vi "Auto Catapult Mode.vi"(9 "Ball Loaded?":bool, 10 "Limit Switch Activated?":bool, 11 "Catapult Commands":T1={"Command"=enum."Prime Shooter", "Mode"=enum."Manual", "Override Trigger Sensor"=FALSE, "High Power Shot?"=FALSE, "Vision?"=FALSE}) -> (0 "Secure Ball?":bool, 1 "Pinned?":bool, 2 "Low Power Solenoid":bool, 3 "High Power Solenoid":bool)   [LabVIEW 2015]
uses:
  Common Code/Catapult/Catapult Command Cluster.ctl
  Common Code/Shooter Commands.ctl
  Common Code/Shoot Modes Enum.ctl
  Common Code/Catapult/Catapult State.ctl
  Common Code/Change Detect Boolean.vi
  Common Code/Change Detect Int.vi
  Robot Global Data.vi
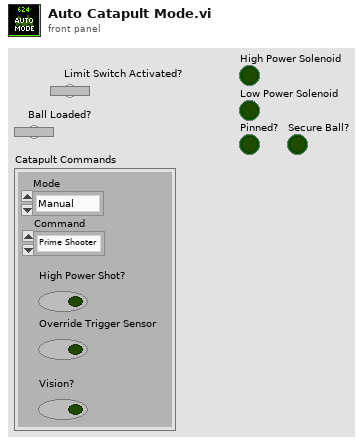
[diagram p1: front panel]
types:
  T1 = typedef "Catapult Command Cluster.ctl" = cluster{"Command":T2, "Mode":T3, "Override Trigger Sensor":bool, "High Power Shot?":bool, "Vision?":bool}
  T2 = typedef "Shooter Commands.ctl" = enum16{"Idle", "Prime Shooter", "Shoot"}
  T3 = typedef "Shoot Modes Enum.ctl" = enum16{"Manual", "Safe", "Auto"}
  T4 = typedef "Catapult State.ctl" = enum16{"Idle", "Warmup", "Shooter Ready", "Shoot"}
  T5 = typedef "Intake Status Cluster.ctl" = cluster{"Roller Power":dbl, "Angle Power":dbl, "Intake Mode":T6, "Intake States":T7, "Rollers Active?":bool, "Current Height":dbl, "Target Height":dbl, "Encoder Raw Position":dbl, "Forward Tripped?":bool, "Backward Tripped?":bool, "Override IR?":bool}
  T6 = typedef "Intake Mode.ctl" = enum16{"Safe", "Auto", "Manual"}
  T7 = typedef "Intake States.ctl" = enum16{"Idle", "Set roller speed", "Move to angle", "Go Hard or Go Home", "Ball Settle"}
  T8 = typedef "Drivetrain Status Cluster.ctl" = cluster{"Modes":T9, "Y (Throttle)":dbl, "X (Steer)":dbl, "Gyro In Range?":bool, "Distance Drive Finished?":bool, "Stop Eject Lockout":bool, "Dist Drive Status":T10, "Y Target":dbl, "Heading Target":dbl, "Vision Target Aligned?":bool, "Gear":dbl, "1st Gear Time":dbl, "2nd Gear Time":dbl, "1st Gear Shifts":dbl, "2nd Gear Shifts":dbl}
  T9 = typedef "Drivetrain Modes.ctl" = enum16{"Tank", "Climb", "Manual", "Goal Vision Targeting", "PID Distance Drive", "Hybrid", "Gyro Steer"}
  T10 = typedef "Dist Drive Status.ctl" = cluster{"Y In Range":bool, "X In Range":bool, "Gyro In Range":bool, "Y Dist":dbl, "X Dist":dbl, "Gyro":dbl}
  T11 = typedef "Dashboard Control Data.ctl" = cluster{"Shooter Presets":T12, "Encoder Control":T14, "Steer PID output":cluster{"output high":dbl, "output low":dbl}, " Steer PID gains":cluster{"proportional gain (Kc)":dbl, "integral time (Ti, min)":dbl, "derivative time (Td, min)":dbl}, "Drivetrain Settings":T15, "Vision Packet":T16, "Dashboard Drivetrain Command":T17, "Info/Command Cluster":T19, "Ball Vision Packet":T20, "Intake Presets":T22, "Intake Encoder Control":T24, "Climb Presets":T25, "Goal Output Range":cluster{"output high":dbl, "output low":dbl}, "Enabled Systems":T26, "Auton Presets":T27, "Pressure M":dbl, "Pressure B":dbl, "Vision Timeout":dbl, "Auto-Shift":T28, "Catapult Setpoints":T29}
  T12 = typedef "Shooter Presets.ctl" = cluster{"Batter Shot":T13, "Deep Middle":T13, "Manual Shot":T13, "Left Ticks Per Rotation":dbl, "Right Ticks Per Rotation":dbl, "Low Bar Shot":T13, "Shooter RPM Tolerance":dbl, "Trigger Power":dbl, "Fire from Load Delay":i32, "Max Angle":dbl, "Min Angle":dbl, "Angle PID gains":cluster{"P":dbl, "I":dbl, "D":dbl}, "Angle Output":cluster{"output high":dbl, "output low":dbl}, "Shooter Angle Tolerance":dbl, "Vision Shoot x^2":dbl, "Vision Shoot x":dbl, "Feed Forward Max Accel":dbl, "Feed Forward Kv":dbl, "Backwards Trigger":dbl, "Shot Finish Delay (ms)":dbl, "Angle Max Current":dbl, "Angle Current Trip Time":dbl, "Intake Angle":dbl, "Vision Shoot c":dbl, "Reset?":bool, "Button Release Delay":dbl, "Angle Pot x":dbl, "Angle Pot c":dbl, "Ignore Angle?":bool, "Max RPM":dbl, "Safty Frist Angle":dbl, "Intake Danger Height":dbl, "Angle Pot B":i32, "Angle Pot M":dbl, "FF Finish RPM":dbl, "RPM PID Right":cluster{"P":dbl, "I":dbl, "D":dbl, "FF":dbl}, "RPM PID Left":cluster{"P":dbl, "I":dbl, "D":dbl, "FF":dbl}, "Backwards RPM":dbl, "Vision RPM":dbl, "Run Wheels Backward Delay":u32, "Cleat Shot":T13, "Vision Far RPM":dbl, "Vision Far Distance":dbl, "Vision Far Angle":dbl}
  T13 = typedef "Shot Presets.ctl" = cluster{"L":dbl, "R":dbl, "A":dbl}
  T14 = typedef "Encoder Control.ctl" = cluster{"Right Tick Constant":dbl, "Left Tick Constant":dbl, "Reset?":bool, "Y Dist":cluster{"PID gains":cluster{"proportional gain (Kc)":dbl, "integral time (Ti, min)":dbl, "derivative time (Td, min)":dbl}}, "Y Stop Thresh":dbl, "Y Stop Speed":dbl}
  T15 = typedef "Drivetrain Settings.ctl" = cluster{"Gyro Tolerance":dbl, "Throttle Ramp (ms)":dbl, "Kv":dbl, "Ka":dbl, "Feed Forward P":dbl, "Feed Forward D":dbl, "Goal Vision PID gains":cluster{"proportional gain (Kc)":dbl, "integral time (Ti, min)":dbl, "derivative time (Td, min)":dbl}, "Goal Detection Window":dbl, "Creep Rate":dbl, "Vision Throttle Threshold":dbl, "Min Turn Output":dbl, "Left Batter Angle":dbl, "Right Batter Angle":dbl}
  T16 = typedef "Goal Vision Packet.ctl" = cluster{"Distance":dbl, "Center X":dbl, "Center Y":dbl, "Found Target?":bool, "Robot Center":dbl, "Angle":dbl}
  T17 = typedef "Dashboard Drivetrain Command.ctl" = cluster{"Drivetrain Vision":T18}
  T18 = typedef "Drivetrain Vision.ctl" = cluster{"Goal Window":dbl, "Ball Window":dbl}
  T19 = typedef "Ball Tracking Command Cluster.ctl" = cluster{"Distance to Ball":dbl, "Desired Angle":dbl, "Command":enum16{"Turn to Ball", "Turn to Angle", "Get Distance"}, "Pixels from Center":dbl}
  T20 = typedef "Ball Vision Packet.ctl" = cluster{"Ball Detected?":bool, "Distance to Ball":dbl, "Desired Angle":dbl, "Pixels from Center":dbl, "Tracking mode":T21}
  T21 = typedef "Tracking Mode.ctl" = enum16{"Turn to Ball", "Turn to Angle"}
  T22 = typedef "Intake Presets.ctl" = cluster{"Intake Speed":dbl, "Outake Speed":dbl, "Low Height":dbl, "Half Height":dbl, "High Idle Height":dbl, "Angle Speed":dbl, "Angle Tolerance":dbl, "Encoder Scale":dbl, "Load Height":dbl, "Output Range":T23, "Rotation Power Max/Min":dbl, "MaxCurrent":dbl, "Intake Trip Time":dbl, "Idle Height":dbl, "Max Height":dbl, "Reset Encoders?":bool, "PID gains":cluster{"proportional gain (Kc)":dbl, "integral time (Ti, min)":dbl, "derivative time (Td, min)":dbl}, "Intake Stop Delay":u32, "Settle Time":dbl, "Settle Wait Time":dbl, "Pull Up Delay":dbl}
  T23 = typedef "Drivetrain Output Range.ctl" = cluster{"output high":dbl, "output low":dbl}
  T24 = typedef "IntakeEcoderControl.ctl" = cluster{"Arm Tick Constant":dbl, "Reset?":bool, "Y Dist":cluster{"PID gains":cluster{"proportional gain (Kc)":dbl, "integral time (Ti, min)":dbl, "derivative time (Td, min)":dbl}}, "Y Stop Thresh":dbl, "Y Stop Speed":dbl}
  T25 = typedef "Climb Presets.ctl" = cluster{"Pull Power":dbl, "Extend Power":dbl}
  T26 = typedef "Enabled Systems.ctl" = cluster{"Shoot":bool, "Intake":bool, "DT":bool, "Gyro":bool, "100ms":bool, "US":bool}
  T27 = typedef "Autonomous Presets.ctl" = cluster{"Pitch Limit":dbl, "Roll Limit":dbl, "Start Position":dbl, "Cross Position":dbl}
  T28 = typedef "Auto Shift Cluster.ctl" = cluster{"Delay":dbl, "Speed Thresh":dbl, "Upshift Accel":dbl, "Upshift Throttle":dbl, "Upshift Throttle Accel":dbl, "Downshift Throttle":dbl, "Downshift Throttle Accel":dbl, "Pressure Threshold":dbl}
  T29 = typedef "Catapult Setpoints.ctl" = cluster{"Intake Danger Height":dbl, "Claw Release Delay":dbl, "Shot Finish Delay":dbl, "Limit Switch Pin Delay":dbl}
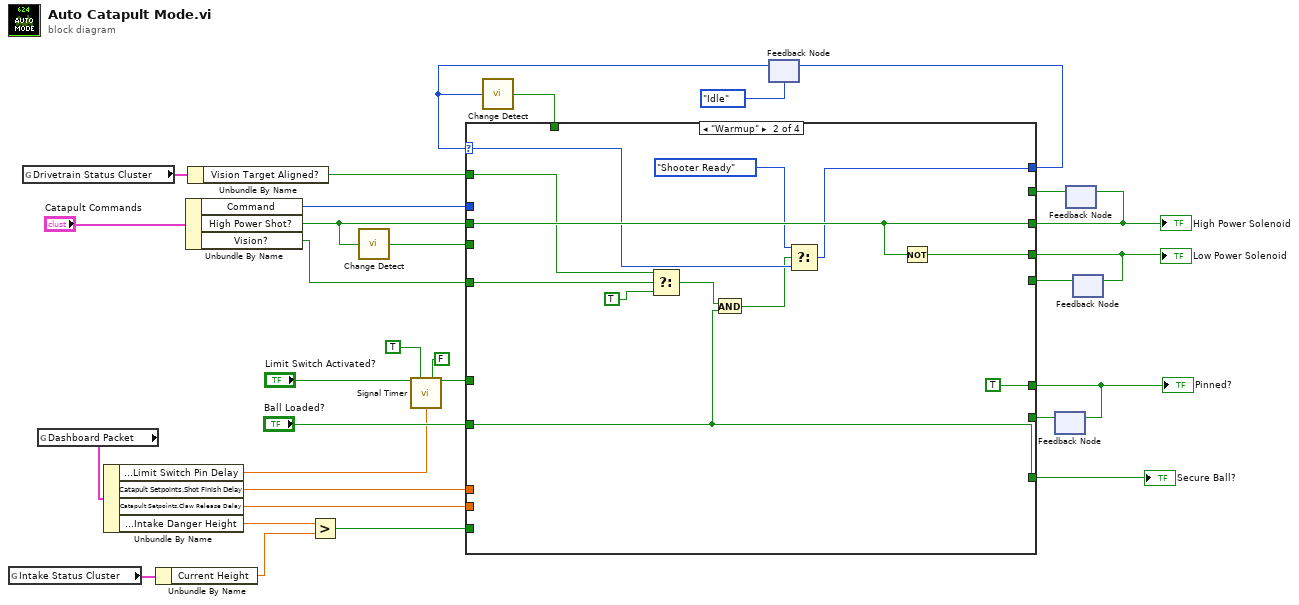
[diagram p0: block diagram]
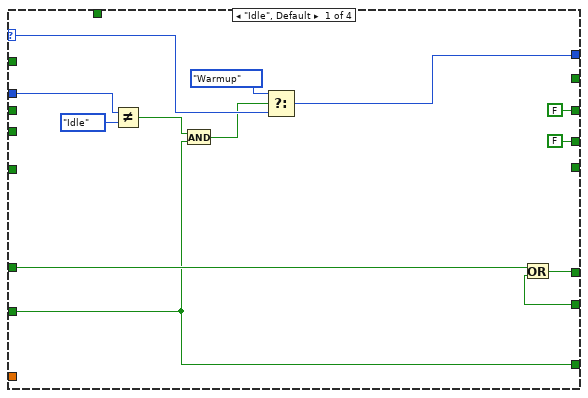
[diagram p2: hidden frame]
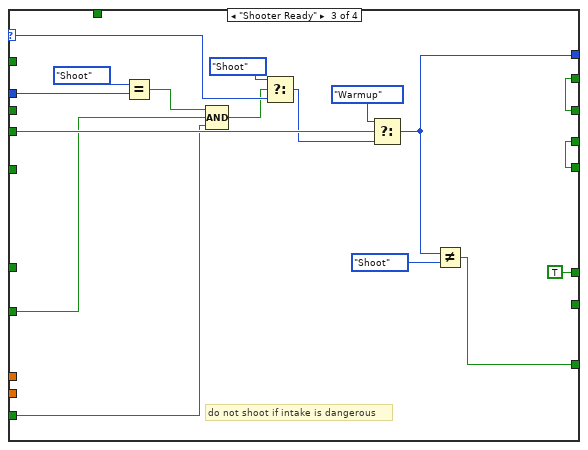
[diagram p3: hidden frame]
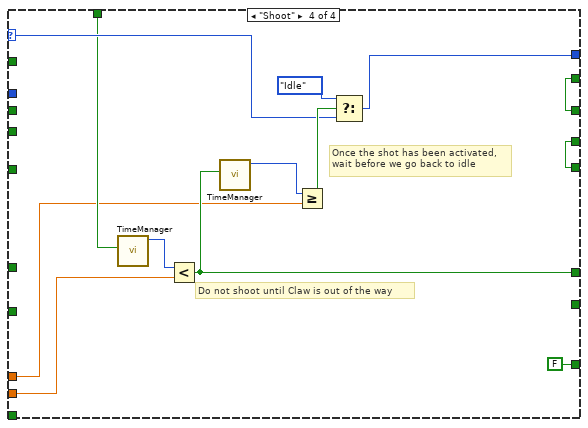
[diagram p4: hidden frame]
diagram:
  n1 = global read "Robot Global Data.vi" "Intake Status Cluster"() -> (w5:T5)
  n2 = global read "Robot Global Data.vi" "Drivetrain Status Cluster"() -> (w13:T8)
  n3 = global read "Robot Global Data.vi" "Dashboard Packet"() -> (w9:T11)
  n4 = Unbundle By Name(w9) -> ("Catapult Setpoints.Limit Switch Pin Delay"=w8:dbl, "Catapult Setpoints.Shot Finish Delay"=w7:dbl, "Catapult Setpoints.Claw Release Delay"=w6:dbl, "Catapult Setpoints.Intake Danger Height"=w4:dbl)
  n5 = Unbundle By Name(w5) -> ("Current Height"=w3:dbl)
  n6 = Unbundle By Name("Catapult Commands") -> ("Command"=w31:T2, "High Power Shot?"=w18:bool, "Vision?"=w14:bool)
  n7 = Unbundle By Name(w13) -> ("Vision Target Aligned?"=w12:bool)
  n8 = Greater?(x=w4, y=w3) -> (0:w2:bool)
  n9 = call-poly "Change Detect.vi"("In"=w18) -> ("Changed?"=w17:bool)
  n10 = call "Signal Timer.vi"("Input"="Limit Switch Activated?", "Edge"=TRUE, "Interval"=w8, "Pull"=FALSE) -> ("Filtered Output"=w21:bool)  [unwired: 11 in]
  n11 = feedback #1(Catapult_State."Idle") -> (w16:T4)
  n12 = call-poly "Change Detect.vi"("In"=w16) -> ("Changed?"=w15:bool)
  n13 = feedback #2() -> (w19:bool)  [unwired: 1 in]
  n14 = feedback #3() -> (w25:bool)  [unwired: 1 in]
  n15 = feedback #4() -> (w27:bool)  [unwired: 1 in]
  n16 = case shown="\"Warmup\"" w16 {
    selector: w16 -> [w42 w48 w68 w82]
    tunnel: w31 -> [w44 _ w70 _]
    tunnel: [w40 w49 w63 w80] -> w29
    tunnel: w18 -> [_ w56 _ _]
    tunnel: [FALSE ("High Power Shot?") w56 w71 w86] -> w26
    tunnel: [FALSE w55 w72 w85] -> w28
    tunnel: [w37 TRUE TRUE w75] -> w20
    tunnel: w27 -> [_ _ w72 w85]
    tunnel: w25 -> [_ _ w71 w86]
    tunnel: w21 -> [w35 _ _ _]
    tunnel: w19 -> [w36 _ _ _]
    tunnel: w17 -> [_ _ w66 _]
    tunnel: w15 -> [_ _ _ w77]
    tunnel: w14 -> [_ w53 _ _]
    tunnel: w12 -> [_ w51 _ _]
    tunnel: "Ball Loaded?" -> [w32 w45 w58 _]
    tunnel: [w32 w45 w61 FALSE ("Ball Loaded?")] -> w10
    tunnel: w7 -> [_ _ _ w74]
    tunnel: w6 -> [_ _ _ w76]
    tunnel: w2 -> [_ _ w57 _]
    frame "Idle", Default {
      n17 = Not Equal?(x=w44, y=Shooter_Commands."Idle") -> (x != y?=w34:bool)
      n18 = And(x=w34, y=w32) -> (x .and. y?=w33:bool)
      n19 = Select(t=Catapult_State."Warmup", s=w33, f=w42) -> (s? t:f=w40:T4)
      n20 = Or(x=w35, y=w36) -> (x .or. y?=w37:bool)
    }
    frame "Warmup" {
      n21 = Select(t=w51, s=w53, f=TRUE ("Pull")) -> (s? t:f=w47:bool)
      n22 = And(x=w47, y=w45) -> (x .and. y?=w46:bool)
      n23 = Select(t=Catapult_State."Shooter Ready", s=w46, f=w48) -> (s? t:f=w49:T4)
      n24 = Not(x=w56) -> (.not. x?=w55:bool)
    }
    frame "Shooter Ready" {
      # "do not shoot if intake is dangerous"
      n25 = Equal?(x=Shooter_Commands."Shoot", y=w70) -> (x = y?=w60:bool)
      n26 = Compound Arithmetic op=AND(w60, w58, w57) -> (w59:bool)
      n27 = Select(t=Catapult_State."Shoot", s=w59, f=w68) -> (s? t:f=w65:T4)
      n28 = Select(t=Catapult_State."Warmup", s=w66, f=w65) -> (s? t:f=w63:T4)
      n29 = Not Equal?(x=w63, y=Catapult_State."Shoot") -> (x != y?=w61:bool)
    }
    frame "Shoot" {
      # "Once the shot has been activated,\nwait before we go back to idle"
      # "Do not shoot until Claw is out of the way"
      n30 = call "TimeManager.vi"("Reset?"=w77) -> ("Time Since Reset"=w78:u32)  [unwired: 9 in, 1 out]
      n31 = Less?(x=w78, y=w76) -> (x < y?=w75:bool)
      n32 = call "TimeManager.vi"("Reset?"=w75) -> ("Time Since Reset"=w84:u32)  [unwired: 9 in, 1 out]
      n33 = Greater Or Equal?(x=w84, y=w74) -> (x >= y?=w83:bool)
      n34 = Select(t=Catapult_State."Idle", s=w83, f=w82) -> (s? t:f=w80:T4)
    }
  }
  "High Power Solenoid" <- w26
  "Low Power Solenoid" <- w28
  "Pinned?" <- w20
  "Secure Ball?" <- w10
  n35 = feedback-in #1(w29) -> ()
  n36 = feedback-in #2(w20) -> ()
  n37 = feedback-in #3(w26) -> ()
  n38 = feedback-in #4(w28) -> ()
